vi "Send Data to ESP32.vi"() -> ()   [LabVIEW 2018]
panel:
  out "Value sent":i32
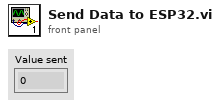
[diagram p1: front panel]
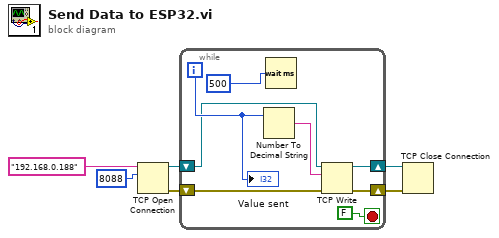
[diagram p0: block diagram]
diagram:
  n1 = TCP Open Connection(address="192.168.0.188", remote port or service name=u16 8088) -> (connection ID=w3:refnum<k5>, error out=w2:errorcluster)  [unwired: 3 in]
  n2 = while {
    shift-right: [w8] -> w6
    shift-left: w3 -> [w10]
    shift-right: [w7] -> w1
    shift-left: w2 -> [w9]
    i -> [w13]
    stop <- FALSE stop-if-true
    n3 = Number To Decimal String(number=w13) -> (decimal integer string=w11:string)  [unwired: 1 in]
    n4 = Wait (ms)(milliseconds to wait=u32 500) -> ()  [unwired: 1 out]
    n5 = TCP Write(connection ID=w10, data in=w11, error in (no error)=w9) -> (connection ID out=w8:refnum<k5>, error out=w7:errorcluster)  [unwired: 1 in, 1 out]
    "Value sent" <- w13
  }
  n6 = TCP Close Connection(connection ID=w6, error in (no error)=w1) -> ()  [unwired: 3 out]
